vi "IMAQ-MWT (FPGA) without PA.vi"() -> ()   [LabVIEW 2015]
uses:
  Modules/Common/Controls (FPGA)/Camera Tap Configuration.ctl
  Modules/Common/Controls (FPGA)/Run Mode.ctl
  <vilib>/Platform/TimedLoop/XDataNode/timing_clust.ctl
  <vilib>/Platform/TimedLoop/XDataNode/nitl_modes.ctl
  <vilib>/Platform/TimedLoop/XDataNode/wakeup.ctl
  Modules/Common/Controls (FPGA)/CL Configuration.ctl
  Modules/Common/Controls (FPGA)/CL Signal Mapping.ctl
  Modules/Common/Controls (FPGA)/Pixel Bundle 40 Bytes.ctl
  <vilib>/rvi/eio/common/nirviEmuTemplateMethod_errors.vi
  <vilib>/rvi/Emulation/niFpgaSctlEmulationGetInTimedLoop.vi
  <vilib>/rvi/Emulation/niFpgaEmulationReportErrorSimple.vi
  <vilib>/rvi/Emulation/niFpgaGetClockAttributes.vi
  <vilib>/rvi/Emulation/niFpgaCriticalErrorInLSC.vi
  Modules/CL Data to Pixels/8 Tap 8-Bit.vi
  Modules/CL Data to Pixels/10 Tap 8-Bit.vi
  <vilib>/rvi/Emulation/niFpgaEmulationIsFPGAContextNoSignature.vi
  <vilib>/rvi/errors/niFpgaSetErrorForExecOnDevCompSimple.vi
  <vilib>/rvi/eio/common/nirviEmuReportErrorAndStop.vi
  <vilib>/rvi/DataTransferAndStorage/Container/Common/niFpgaContainerGetUniqueNameForEmu.vi
  <vilib>/rvi/FIFO/Fifo_Resource/nirvififoEmulationSetSize.vi
  <vilib>/rvi/FIFO/Fifo_Resource/nirviFifoEmulationQueueMgr.vi
  <instcachedir>/0/nirviFifoEmulationQueueMgr_E5CAEC123FF24DC58D834DCA3CDAA9B5.lvgen/nirviFifoEmulationQueueMgr_E5CAEC123FF24DC58D834DCA3CDAA9B5_008.vi
  <vilib>/rvi/FIFO/Fifo_Resource/nirvififoEmulationDetermineInputValidOut.vi
  <vilib>/rvi/FIFO/Fifo_Resource/nirvififoEmulationCreateLock.vi
  <vilib>/rvi/Emulation/niFpgaProcessEmulError.vi
  <vilib>/rvi/FIFO/Fifo_Resource/nirvififoEmulationObtainLock.vi
  <vilib>/rvi/FIFO/Fifo_Resource/nirvififoEmulationReleaseLock.vi
  <vilib>/rvi/occurrence/nirviWaitOnOccurrenceBase.vi
  <vilib>/rvi/errors/nirviReportUnexpectedCaseInternalError.vi
  <vilib>/rvi/errors/nirviReportUnexpectedCaseInternalError (U32).vi
  <instcachedir>/0/nirviFifoEmulationQueueMgr_E5CAEC123FF24DC58D834DCA3CDAA9B5.lvgen/nirviFifoEmulationQueueMgr_E5CAEC123FF24DC58D834DCA3CDAA9B5_004.vi
  <vilib>/Utility/error.llb/Clear Errors.vi
  <vilib>/rvi/interface/RandomDataEmulation/niFpgaRandomDataHandleErrors.vi
  <instcachedir>/0/nirviFifoEmulationQueueMgr_E5CAEC123FF24DC58D834DCA3CDAA9B5.lvgen/nirviFifoEmulationQueueMgr_E5CAEC123FF24DC58D834DCA3CDAA9B5_001.vi
  <vilib>/eio/EIONode/EIONode.xnode
  <vilib>/Platform/TimedLoop/XDataNode/XDataNode.xnode
  <vilib>/rvi/DataTransferAndStorage/Container/XNode/niFpgaContainer.xnode
  <vilib>/rvi/FIFO/Fifo_Resource/nirvififoEmulationWrite.vi
  <vilib>/rvi/FIFO/Fifo_Resource/nirvififoEmulationRead.vi
  <vilib>/rvi/interface/RandomDataEmulation/nirviRandomDataFpgaReadWriteTemplate.vi
  <vilib>/Platform/TimedLoop/XDataNode/XDNodeRunTimeDep.lvlib
panel:
  in  "Significant Angle":fxp<+,16,3>=0.0999755859375 format="%#_14g"
  in  "Mode":T1
  out "Frame Interval":u32=4294967295
  out "Frame #":u32
  in  "Image Height":u16=3072
  in  "Image Width":u16=3072
  out "PoCL Power Is On":bool
  in  "N Spline Points":fxp<+,8,8>=31.0
  in  "Clock Cycles Limit":u32=10000
  in  "Pixel Intensity":cluster{"Low":u8, "High":u8}={"Low"=100, "High"=255}
  out "DMA Timeout":bool
  in  "Cancel Acq":bool
  in  "Acquire":bool
  out "Acq In Progress":bool
  in  "Tap Configuration":T2
  in  "Initialize":bool=TRUE
  out "Initialized":bool=TRUE
  # "IMAQ - MWT"
  # "Camera Link Configuration"
  # "Acquisition Settings"
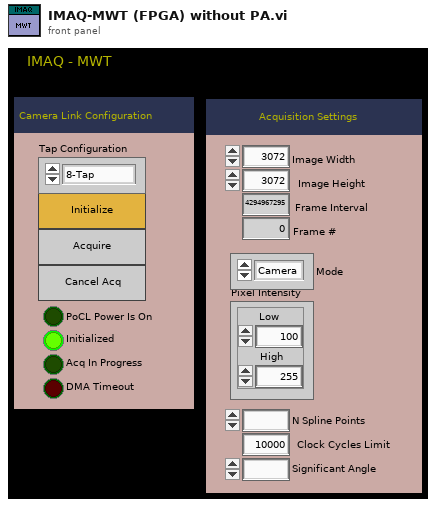
[diagram p1: front panel]
types:
  T1 = typedef "Run Mode.ctl" = enum16{"Camera", "Video (Raw)", "Video (DBDE)"}
  T2 = typedef "Camera Tap Configuration.ctl" = enum8{"8-Tap", "10-Tap"}
  T3 = typedef "CL Signal Mapping.ctl" = enum8{"Standard", "Basler 10-tap", "Vosskühler 10-tap"}
  T4 = typedef "CL Configuration.ctl" = enum8{"Base", "Medium", "Full"}
  T5 = typedef "XDNodeRunTimeDep.lvlib/timing_clust.ctl" = cluster{"Expected End [f-1]":u64, "Actual End [f-1]":u64, "Finished Late? [f-1]":bool, "Expected End [i-1]":u64, "Actual End [i-1]":u64, "Finished Late? [i-1]":bool, "Expected Start [i]":u64, "Actual Start [i]":u64, "Expected Start [f]":u64, "Actual Start [f]":u64, "Source Name":string, "Structure Name":string, "Period":i64, "Deadline":i64, "Offset":i64, "Start":i64, "Priority":i32, "Timeout":i32, "Mode":T6, "Wakeup Reason":T7, "Error":errorcluster, "Source Type":string, "Secondary Source Type":string, "Global End Time":u64, "Global Start Time":u64, "Frame Duration":u64, "Iteration Duration":u64, "Assigned CPU":i32, "I/O Scan Engine Mode":u32}
  T6 = typedef "XDNodeRunTimeDep.lvlib/nitl_modes.ctl" = enum32{"No Change", "Process missed periods, maintain original phase", "Discard missed periods, maintain original phase", "Process missed periods, ignore original phase", "Discard missed periods, ignore original phase"}
  T7 = typedef "XDNodeRunTimeDep.lvlib/wakeup.ctl" = enum32{"Normal", "Aborted", "Asynchronous wakeup", "Timing source error", "Timed loop error", "Timeout"}
  T8 = typedef "Pixel Bundle 40 Bytes.ctl" = cluster{"Pixel 1":u8, "Pixel 2":u8, "Pixel 3":u8, "Pixel 4":u8, "Pixel 5":u8, "Pixel 6":u8, "Pixel 7":u8, "Pixel 8":u8, "Pixel 9":u8, "Pixel 10":u8, "Pixel 11":u8, "Pixel 12":u8, "Pixel 13":u8, "Pixel 14":u8, "Pixel 15":u8, "Pixel 16":u8, "Pixel 17":u8, "Pixel 18":u8, "Pixel 19":u8, "Pixel 20":u8, "Pixel 21":u8, "Pixel 22":u8, "Pixel 23":u8, "Pixel 24":u8, "Pixel 25":u8, "Pixel 26":u8, "Pixel 27":u8, "Pixel 28":u8, "Pixel 29":u8, "Pixel 30":u8, "Pixel 31":u8, "Pixel 32":u8, "Pixel 33":u8, "Pixel 34":u8, "Pixel 35":u8, "Pixel 36":u8, "Pixel 37":u8, "Pixel 38":u8, "Pixel 39":u8, "Pixel 40":u8}
  T9 = cluster{"Enables Valid":bool, "Frame Valid":bool, "Line Valid":bool, "Data Valid":bool}
  T10 = cluster{"Pixel 0":u8, "Pixel 1":u8, "Pixel 2":u8, "Pixel 3":u8, "Pixel 4":u8, "Pixel 5":u8, "Pixel 6":u8, "Pixel 7":u8, "Pixel 8":u8, "Pixel 9":u8}
  T11 = cluster{"Pixel 0":u8, "Pixel 1":u8, "Pixel 2":u8, "Pixel 3":u8, "Pixel 4":u8, "Pixel 5":u8, "Pixel 6":u8, "Pixel 7":u8}
  T12 = cluster{"Pixel 1":u8, "Pixel 2":u8, "Pixel 3":u8, "Pixel 4":u8, "Pixel 5":u8, "Pixel 6":u8, "Pixel 7":u8, "Pixel 8":u8, "Pixel 9":u8, "Pixel 10":u8}
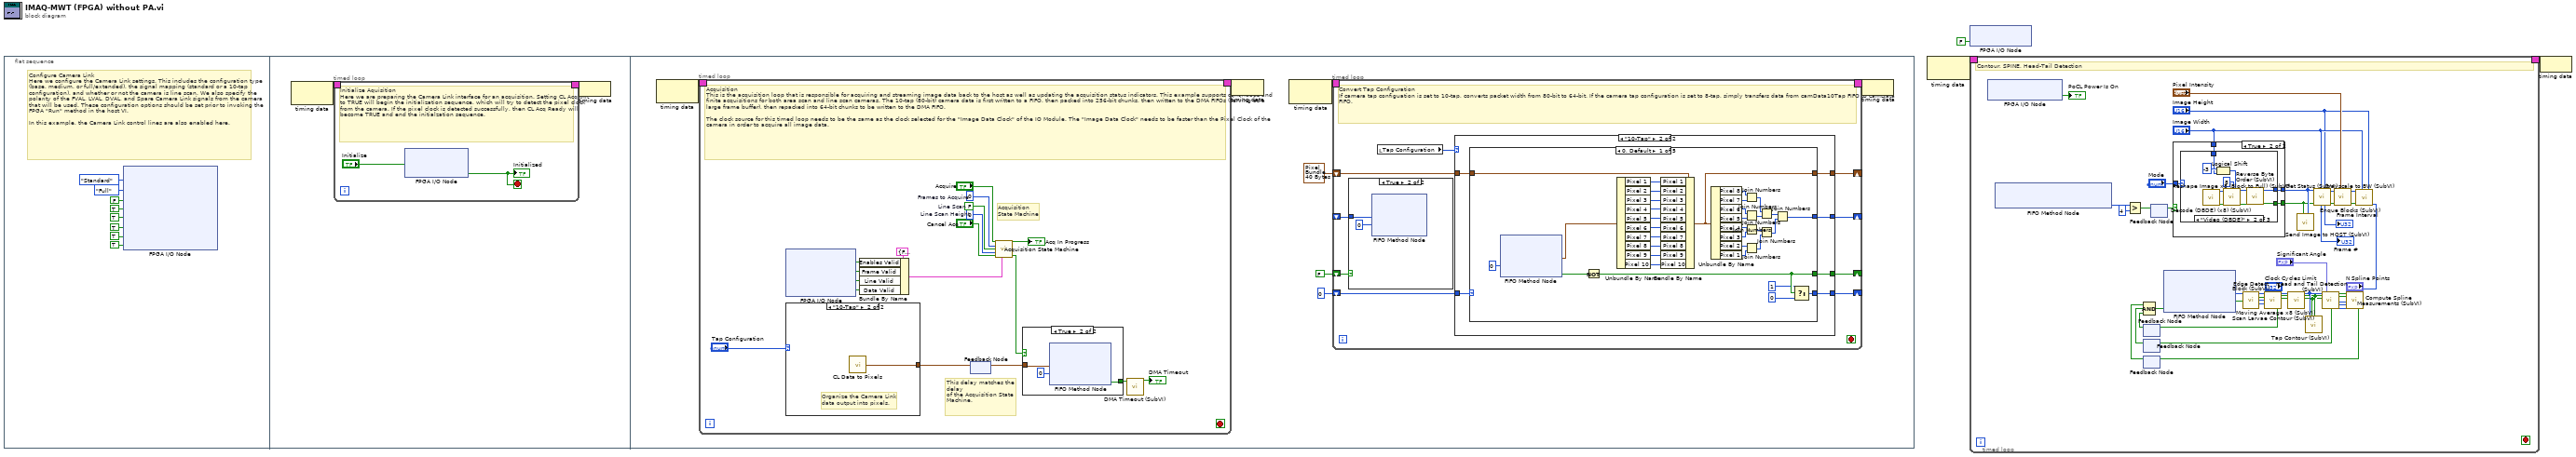
[diagram p0: block diagram]
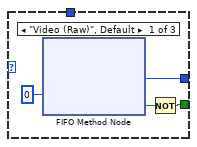
[diagram p3: hidden frame]
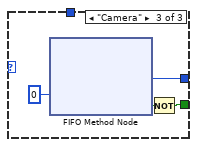
[diagram p4: hidden frame]
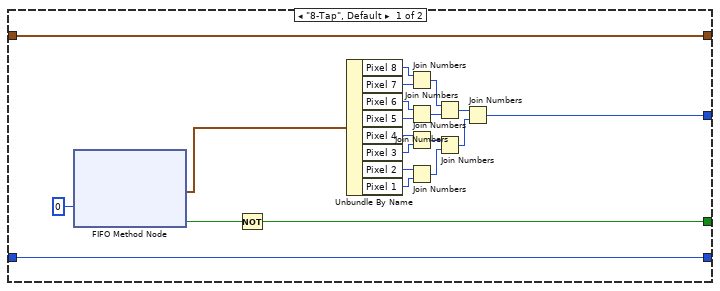
[diagram p6: hidden frame]
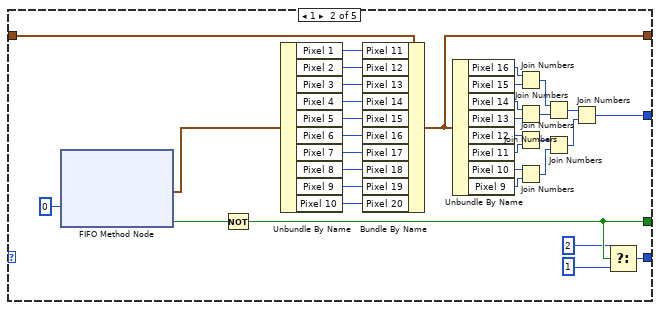
[diagram p7: hidden frame]
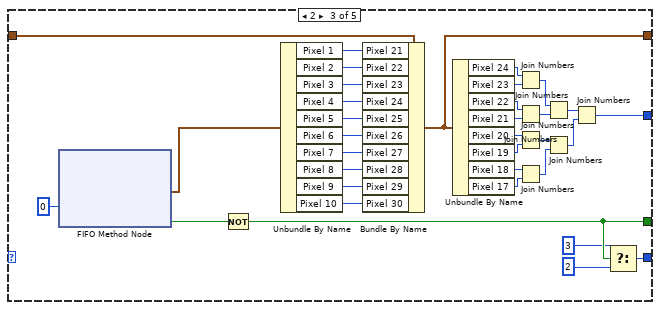
[diagram p8: hidden frame]
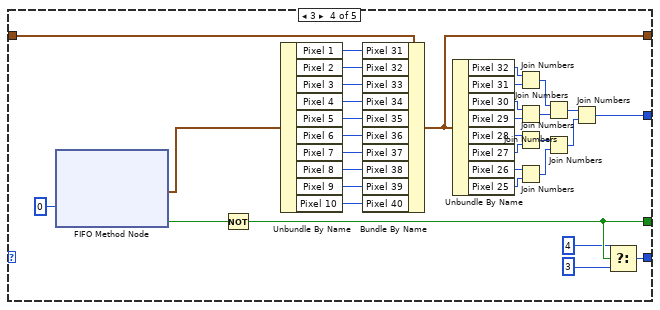
[diagram p9: hidden frame]
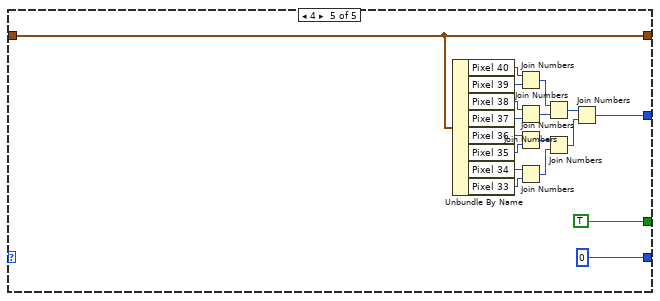
[diagram p10: hidden frame]
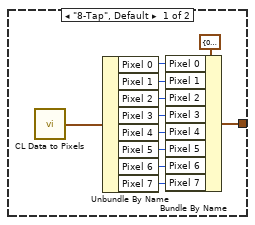
[diagram p11: hidden frame]
diagram:
  n1 = flat-sequence {
    frame #0 {
      # "Configure Camera Link\nHere we configure the Camera Link settings. This includes the configuration type (base, medium, or full/extended), the signal mapping (standard or a 10-tap configuration), and whether or not the camera is line scan. We also specify the polarity of the FVAL, LVAL, DVAL, and Spare Camera Link signals from the camera that will be used. These configuration options should be set prior to invoking the FPGA \"Run\" method in the host VI.\n\nIn this example, the Camera Link control lines are also enabled here."
      n2 = xnode "FPGA I/O Node"("CL Set Configuration"=CL_Signal_Mapping."Standard" ("Signal Mapping"), "CL Set Configuration"=CL_Configuration."Full" ("Configuration"), "CL Set Line Scan"=FALSE ("Line Scan"), "CL Set FVAL Active High"=TRUE ("FVAL Active High"), "CL Set LVAL Active High"=TRUE ("LVAL Active High"), "CL Set DVAL Active High"=TRUE ("DVAL Active High"), "CL Set Spare Active High"=TRUE ("Spare Active High"), "CL Control Enable"=TRUE ("IO Module\\CL Control Enable")) -> ()  [unwired: 8 in, 8 out]
    }
    frame #1 {
      n3 = node-c288() -> (w13:T5)  [unwired: 1 out]
      n4 = timed-loop {
        timing: w13 -> [_]
        timing-out: [_] -> w12
        stop <- w14 stop-if-true
        # "Initialize Aquisition\nHere we are preparing the Camera Link interface for an acquisition. Setting CL Acq Init to TRUE will begin the initialization sequence, which will try to detect the pixel clock from the camera. If the pixel clock is detected successfully, then CL Acq Ready will become TRUE and end the initialzation sequence."
        n5 = xnode "FPGA I/O Node"("CL Acq Init"="Initialize") -> ("CL Acq Ready"=w14:bool)  [unwired: 2 in, 2 out]
        "Initialized" <- w14
      }
      n6 = node-c288(w12) -> ()
    }
    frame #2 {
      n7 = node-c288() -> (w26:T5)  [unwired: 1 in]
      n8 = timed-loop {
        timing: w26 -> [_]
        timing-out: [_] -> w25
        stop <- _ stop-if-true
        w224 = FALSE  # Line Scan
        w225 = u32 0  # Line Scan Height
        w226 = u32 0  # Frames to Acquire
        # "This delay matches the delay\nof the Acquisition State Machine."
        # "Acquisition\nState Machine"
        # "Acquisition\nThis is the acquisition loop that is responsible for acquiring and streaming image data back to the host as well as updating the acquisition status indicators. This example supports continuous and finite acquisitions for both area scan and line scan cameras. The 10-tap (80-bit) camera data is first written to a FIFO, then packed into 256-bit chunks, then written to the DMA FIFOs (serving as a large frame buffer), then repacked into 64-bit chunks to be written to the DMA FIFO. \n\nThe clock source for this timed loop needs to be the same as the clock selected for the \"Image Data Clock\" of the IO Module. The \"Image Data Clock\" needs to be faster than the Pixel Clock of the camera in order to acquire all image data."
        n9 = xnode "FPGA I/O Node"() -> ("CL Output Valid"=w237:bool, "CL Frame Valid"=w236:bool, "CL Line Valid"=w235:bool, "CL Data Valid"=w233:bool)  [unwired: 4 in, 4 out]
        n10 = case shown="\"10-Tap\"" "Tap Configuration" {
          tunnel: [w241 w252] -> w229
          frame "8-Tap", Default {
            n11 = call-poly "CL Data to Pixels.vi"() -> ("Pixels"=w250:T11)  [unwired: 1 in]
            n12 = Unbundle By Name(w250) -> ("Pixel 0"=w249:u8, "Pixel 1"=w248:u8, "Pixel 2"=w247:u8, "Pixel 3"=w246:u8, "Pixel 4"=w245:u8, "Pixel 5"=w244:u8, "Pixel 6"=w243:u8, "Pixel 7"=w242:u8)
            n13 = Bundle By Name(cluster=T10 {"Pixel 0"=0, "Pixel 1"=0, "Pixel 2"=0, "Pixel 3"=0, "Pixel 4"=0, "Pixel 5"=0, "Pixel 6"=0, "Pixel 7"=0, "Pixel 8"=0, "Pixel 9"=0} ("Pixels"), "Pixel 0"=w249, "Pixel 1"=w248, "Pixel 2"=w247, "Pixel 3"=w246, "Pixel 4"=w245, "Pixel 5"=w244, "Pixel 6"=w243, "Pixel 7"=w242) -> (w241:T10)
          }
          frame "10-Tap" {
            # "Organize the Camera Link\ndata output into pixels."
            n14 = call-poly "CL Data to Pixels.vi"() -> ("Pixels"=w252:T10)  [unwired: 1 in]
          }
        }
        n15 = Bundle By Name(cluster=T9 {"Enables Valid"=FALSE, "Frame Valid"=FALSE, "Line Valid"=FALSE, "Data Valid"=FALSE} ("Enables"), "Enables Valid"=w237, "Frame Valid"=w236, "Line Valid"=w235, "Data Valid"=w233) -> (w234:T9)
        n16 = feedback-in #1(w229) -> ()
        n17 = feedback #1() -> (w230:T10)  [unwired: 1 in]
        n18 = call "Acquisition State Machine.vi"("Acquire"="Acquire", "Frames to Acquire"=w226, "Line Scan"=w224, "Line Scan Height"=w225, "Cancel Acq"="Cancel Acq", "Enables"=w234) -> ("Acq In Progress"=→"Acq In Progress":bool, "Capture Cycle"=w231:bool)  [unwired: 4 in, 4 out]
        n19 = case shown="True" w231 {
          tunnel: [_ w253] -> w227
          tunnel: w230 -> [_ w254]
          frame False {
          }
          frame True {
            n20 = xnode ("FIFO Method Node")("Element"=w254, "Timeout"=0) -> ("Timed Out?"=w253:bool)  [unwired: 1 in, 1 out]
          }
        }
        n21 = call "DMA Timeout (SubVI).vi"("Timeout"=w227) -> ("DMA Timeout"=→"DMA Timeout":bool)  [unwired: 10 in]
      }
      n22 = node-c288(w25) -> ()
      n23 = node-c288() -> (w24:T5)  [unwired: 1 in]
      n24 = timed-loop {
        timing: w24 -> [_]
        timing-out: [_] -> w23
        shift-right: [w33] -> _
        shift-left: u8 0 ("Timeout") -> [w34]
        shift-right: [w31] -> _
        shift-left: T8 {"Pixel 1"=0, "Pixel 2"=0, "Pixel 3"=0, "Pixel 4"=0, "Pixel 5"=0, "Pixel 6"=0, "Pixel 7"=0, "Pixel 8"=0, "Pixel 9"=0, "Pixel 10"=0, "Pixel 11"=0, "Pixel 12"=0, "Pixel 13"=0, "Pixel 14"=0, "Pixel 15"=0, "Pixel 16"=0, "Pixel 17"=0, "Pixel 18"=0, "Pixel 19"=0, "Pixel 20"=0, "Pixel 21"=0, "Pixel 22"=0, "Pixel 23"=0, "Pixel 24"=0, "Pixel 25"=0, "Pixel 26"=0, "Pixel 27"=0, "Pixel 28"=0, "Pixel 29"=0, "Pixel 30"=0, "Pixel 31"=0, "Pixel 32"=0, "Pixel 33"=0, "Pixel 34"=0, "Pixel 35"=0, "Pixel 36"=0, "Pixel 37"=0, "Pixel 38"=0, "Pixel 39"=0, "Pixel 40"=0} ("Data In") -> [w32]
        shift-right: [w30] -> _
        shift-left: _ -> [w27]
        shift-right: [w29] -> _
        shift-left: FALSE -> [w28]
        stop <- _ stop-if-true
        # "Convert Tap Configuration\nIf camera tap configuation is set to 10-tap, converts packet width from 80-bit to 64-bit. If the camera tap configuration is set to 8-tap, simply transfers data from camData10Tap FIFO to camData FIFO."
        n25 = case shown="True" w28 {
          tunnel: w27 -> [_ w37]
          frame False {
          }
          frame True {
            n26 = xnode ("FIFO Method Node")("Element"=w37, "Timeout"=0) -> ()  [unwired: 1 in, 2 out]
          }
        }
        n27 = local read "Tap Configuration"() -> (w35:T2)
        n28 = case shown="\"10-Tap\"" w35 {
          tunnel: [w44 w63] -> w29
          tunnel: [w43 w62] -> w30
          tunnel: w34 -> [w42 w64]
          tunnel: [w42 w61] -> w33
          tunnel: w32 -> [w41 w60]
          tunnel: [w41 w59] -> w31
          frame "8-Tap", Default {
            n29 = xnode ("FIFO Method Node")("Timeout"=0) -> ("Element"=w40:T12, "Timed Out?"=w39:bool)  [unwired: 1 in, 1 out]
            n30 = Not(x=w39) -> (.not. x?=w44:bool)
            n31 = Unbundle By Name(w40) -> ("Pixel 8"=w58:u8, "Pixel 7"=w57:u8, "Pixel 6"=w56:u8, "Pixel 5"=w55:u8, "Pixel 4"=w53:u8, "Pixel 3"=w54:u8, "Pixel 2"=w51:u8, "Pixel 1"=w52:u8)
            n32 = Join Numbers(hi=w58, lo=w57) -> ((hi.lo)=w49:u16)
            n33 = Join Numbers(hi=w56, lo=w55) -> ((hi.lo)=w50:u16)
            n34 = Join Numbers(hi=w53, lo=w54) -> ((hi.lo)=w48:u16)
            n35 = Join Numbers(hi=w51, lo=w52) -> ((hi.lo)=w47:u16)
            n36 = Join Numbers(hi=w49, lo=w50) -> ((hi.lo)=w46:u32)
            n37 = Join Numbers(hi=w48, lo=w47) -> ((hi.lo)=w45:u32)
            n38 = Join Numbers(hi=w46, lo=w45) -> ((hi.lo)=w43:u64)
          }
          frame "10-Tap" {
            n39 = case shown="0, Default" w64 {
              tunnel: [w82 w116 w150 w184 TRUE] -> w63
              tunnel: [w84 w118 w152 w186 w204] -> w62
              tunnel: [w83 w117 w151 w185 u8 0 ("Timeout")] -> w61
              tunnel: w60 -> [w79 w113 w147 w181 w203]
              tunnel: [w78 w112 w146 w180 w203] -> w59
              frame 0, Default {
                n40 = xnode ("FIFO Method Node")("Timeout"=0) -> ("Element"=w66:T12, "Timed Out?"=w67:bool)  [unwired: 1 in, 1 out]
                n41 = Not(x=w67) -> (.not. x?=w82:bool)
                n42 = Unbundle By Name(w66) -> ("Pixel 1"=w77:u8, "Pixel 2"=w76:u8, "Pixel 3"=w75:u8, "Pixel 4"=w74:u8, "Pixel 5"=w73:u8, "Pixel 6"=w72:u8, "Pixel 7"=w71:u8, "Pixel 8"=w70:u8, "Pixel 9"=w69:u8, "Pixel 10"=w68:u8)
                n43 = Bundle By Name(cluster=w79, "Pixel 1"=w77, "Pixel 2"=w76, "Pixel 3"=w75, "Pixel 4"=w74, "Pixel 5"=w73, "Pixel 6"=w72, "Pixel 7"=w71, "Pixel 8"=w70, "Pixel 9"=w69, "Pixel 10"=w68) -> (w78:T8)
                n44 = Unbundle By Name(w78) -> ("Pixel 8"=w98:u8, "Pixel 7"=w97:u8, "Pixel 6"=w96:u8, "Pixel 5"=w95:u8, "Pixel 4"=w93:u8, "Pixel 3"=w94:u8, "Pixel 2"=w91:u8, "Pixel 1"=w92:u8)
                n45 = Join Numbers(hi=w98, lo=w97) -> ((hi.lo)=w89:u16)
                n46 = Join Numbers(hi=w96, lo=w95) -> ((hi.lo)=w90:u16)
                n47 = Join Numbers(hi=w93, lo=w94) -> ((hi.lo)=w88:u16)
                n48 = Join Numbers(hi=w91, lo=w92) -> ((hi.lo)=w87:u16)
                n49 = Join Numbers(hi=w89, lo=w90) -> ((hi.lo)=w86:u32)
                n50 = Join Numbers(hi=w88, lo=w87) -> ((hi.lo)=w85:u32)
                n51 = Join Numbers(hi=w86, lo=w85) -> ((hi.lo)=w84:u64)
                n52 = Select(t=u8 1 ("Timeout"), s=w82, f=u8 0 ("Timeout")) -> (s? t:f=w83:u8)
              }
              frame 1 {
                n53 = xnode ("FIFO Method Node")("Timeout"=0) -> ("Element"=w101:T12, "Timed Out?"=w100:bool)  [unwired: 1 in, 1 out]
                n54 = Not(x=w100) -> (.not. x?=w116:bool)
                n55 = Unbundle By Name(w101) -> ("Pixel 1"=w111:u8, "Pixel 2"=w110:u8, "Pixel 3"=w109:u8, "Pixel 4"=w108:u8, "Pixel 5"=w107:u8, "Pixel 6"=w106:u8, "Pixel 7"=w105:u8, "Pixel 8"=w104:u8, "Pixel 9"=w103:u8, "Pixel 10"=w102:u8)
                n56 = Bundle By Name(cluster=w113, "Pixel 11"=w111, "Pixel 12"=w110, "Pixel 13"=w109, "Pixel 14"=w108, "Pixel 15"=w107, "Pixel 16"=w106, "Pixel 17"=w105, "Pixel 18"=w104, "Pixel 19"=w103, "Pixel 20"=w102) -> (w112:T8)
                n57 = Unbundle By Name(w112) -> ("Pixel 16"=w132:u8, "Pixel 15"=w131:u8, "Pixel 14"=w130:u8, "Pixel 13"=w129:u8, "Pixel 12"=w127:u8, "Pixel 11"=w128:u8, "Pixel 10"=w125:u8, "Pixel 9"=w126:u8)
                n58 = Join Numbers(hi=w132, lo=w131) -> ((hi.lo)=w123:u16)
                n59 = Join Numbers(hi=w130, lo=w129) -> ((hi.lo)=w124:u16)
                n60 = Join Numbers(hi=w127, lo=w128) -> ((hi.lo)=w122:u16)
                n61 = Join Numbers(hi=w125, lo=w126) -> ((hi.lo)=w121:u16)
                n62 = Join Numbers(hi=w123, lo=w124) -> ((hi.lo)=w120:u32)
                n63 = Join Numbers(hi=w122, lo=w121) -> ((hi.lo)=w119:u32)
                n64 = Join Numbers(hi=w120, lo=w119) -> ((hi.lo)=w118:u64)
                n65 = Select(t=u8 2 ("Timeout"), s=w116, f=u8 1 ("Timeout")) -> (s? t:f=w117:u8)
              }
              frame 2 {
                n66 = xnode ("FIFO Method Node")("Timeout"=0) -> ("Element"=w134:T12, "Timed Out?"=w135:bool)  [unwired: 1 in, 1 out]
                n67 = Not(x=w135) -> (.not. x?=w150:bool)
                n68 = Unbundle By Name(w134) -> ("Pixel 1"=w145:u8, "Pixel 2"=w144:u8, "Pixel 3"=w143:u8, "Pixel 4"=w142:u8, "Pixel 5"=w141:u8, "Pixel 6"=w140:u8, "Pixel 7"=w139:u8, "Pixel 8"=w138:u8, "Pixel 9"=w137:u8, "Pixel 10"=w136:u8)
                n69 = Bundle By Name(cluster=w147, "Pixel 21"=w145, "Pixel 22"=w144, "Pixel 23"=w143, "Pixel 24"=w142, "Pixel 25"=w141, "Pixel 26"=w140, "Pixel 27"=w139, "Pixel 28"=w138, "Pixel 29"=w137, "Pixel 30"=w136) -> (w146:T8)
                n70 = Unbundle By Name(w146) -> ("Pixel 24"=w166:u8, "Pixel 23"=w165:u8, "Pixel 22"=w164:u8, "Pixel 21"=w163:u8, "Pixel 20"=w161:u8, "Pixel 19"=w162:u8, "Pixel 18"=w159:u8, "Pixel 17"=w160:u8)
                n71 = Join Numbers(hi=w166, lo=w165) -> ((hi.lo)=w157:u16)
                n72 = Join Numbers(hi=w164, lo=w163) -> ((hi.lo)=w158:u16)
                n73 = Join Numbers(hi=w161, lo=w162) -> ((hi.lo)=w156:u16)
                n74 = Join Numbers(hi=w159, lo=w160) -> ((hi.lo)=w155:u16)
                n75 = Join Numbers(hi=w157, lo=w158) -> ((hi.lo)=w154:u32)
                n76 = Join Numbers(hi=w156, lo=w155) -> ((hi.lo)=w153:u32)
                n77 = Join Numbers(hi=w154, lo=w153) -> ((hi.lo)=w152:u64)
                n78 = Select(t=u8 3 ("Timeout"), s=w150, f=u8 2 ("Timeout")) -> (s? t:f=w151:u8)
              }
              frame 3 {
                n79 = xnode ("FIFO Method Node")("Timeout"=0) -> ("Element"=w168:T12, "Timed Out?"=w169:bool)  [unwired: 1 in, 1 out]
                n80 = Not(x=w169) -> (.not. x?=w184:bool)
                n81 = Unbundle By Name(w168) -> ("Pixel 1"=w179:u8, "Pixel 2"=w178:u8, "Pixel 3"=w177:u8, "Pixel 4"=w176:u8, "Pixel 5"=w175:u8, "Pixel 6"=w174:u8, "Pixel 7"=w173:u8, "Pixel 8"=w172:u8, "Pixel 9"=w171:u8, "Pixel 10"=w170:u8)
                n82 = Bundle By Name(cluster=w181, "Pixel 31"=w179, "Pixel 32"=w178, "Pixel 33"=w177, "Pixel 34"=w176, "Pixel 35"=w175, "Pixel 36"=w174, "Pixel 37"=w173, "Pixel 38"=w172, "Pixel 39"=w171, "Pixel 40"=w170) -> (w180:T8)
                n83 = Unbundle By Name(w180) -> ("Pixel 32"=w200:u8, "Pixel 31"=w199:u8, "Pixel 30"=w198:u8, "Pixel 29"=w197:u8, "Pixel 28"=w195:u8, "Pixel 27"=w196:u8, "Pixel 26"=w193:u8, "Pixel 25"=w194:u8)
                n84 = Join Numbers(hi=w200, lo=w199) -> ((hi.lo)=w191:u16)
                n85 = Join Numbers(hi=w198, lo=w197) -> ((hi.lo)=w192:u16)
                n86 = Join Numbers(hi=w195, lo=w196) -> ((hi.lo)=w190:u16)
                n87 = Join Numbers(hi=w193, lo=w194) -> ((hi.lo)=w189:u16)
                n88 = Join Numbers(hi=w191, lo=w192) -> ((hi.lo)=w188:u32)
                n89 = Join Numbers(hi=w190, lo=w189) -> ((hi.lo)=w187:u32)
                n90 = Join Numbers(hi=w188, lo=w187) -> ((hi.lo)=w186:u64)
                n91 = Select(t=u8 4 ("Timeout"), s=w184, f=u8 3 ("Timeout")) -> (s? t:f=w185:u8)
              }
              frame 4 {
                n92 = Unbundle By Name(w203) -> ("Pixel 40"=w218:u8, "Pixel 39"=w217:u8, "Pixel 38"=w216:u8, "Pixel 37"=w215:u8, "Pixel 36"=w213:u8, "Pixel 35"=w214:u8, "Pixel 34"=w211:u8, "Pixel 33"=w212:u8)
                n93 = Join Numbers(hi=w218, lo=w217) -> ((hi.lo)=w209:u16)
                n94 = Join Numbers(hi=w216, lo=w215) -> ((hi.lo)=w210:u16)
                n95 = Join Numbers(hi=w213, lo=w214) -> ((hi.lo)=w208:u16)
                n96 = Join Numbers(hi=w211, lo=w212) -> ((hi.lo)=w207:u16)
                n97 = Join Numbers(hi=w209, lo=w210) -> ((hi.lo)=w206:u32)
                n98 = Join Numbers(hi=w208, lo=w207) -> ((hi.lo)=w205:u32)
                n99 = Join Numbers(hi=w206, lo=w205) -> ((hi.lo)=w204:u64)
              }
            }
          }
        }
      }
      n100 = node-c288(w23) -> ()
    }
  }
  n101 = node-c288() -> (w3:T5)  [unwired: 1 in]
  n102 = xnode "FPGA I/O Node"("PoCL Disable"=FALSE) -> ()  [unwired: 1 in, 1 out]
  n103 = timed-loop {
    timing: w3 -> [_]
    timing-out: [_] -> w2
    stop <- _ stop-if-true
    # "Contour, SPINE, Head-Tail Detection"
    n104 = xnode "FPGA I/O Node"() -> ("PoCL Power Is On"=→"PoCL Power Is On":bool)  [unwired: 1 in, 1 out]
    n105 = xnode ("FIFO Method Node")() -> ("Number of Elements to Write"=w285:u32)  [unwired: 1 in, 1 out]
    n106 = Greater?(x=w285, y=u32 4) -> (0:w289:bool)
    n107 = feedback #2() -> (w292:bool)  [unwired: 1 in]
    n108 = feedback #3() -> (w293:bool)  [unwired: 1 in]
    n109 = feedback #4() -> (w291:bool)  [unwired: 1 in]
    n110 = Compound Arithmetic op=AND(w291, w293, w292) -> (w284:bool)
    n111 = feedback-in #5(w289) -> ()
    n112 = feedback #5() -> (w288:bool)  [unwired: 1 in]
    n113 = xnode ("FIFO Method Node")("Ready for Output"=w284) -> ("Element"=w283:u8, "Output Valid"=w282:bool)  [unwired: 1 in, 1 out]
    n114 = case shown="True" w288 {
      tunnel: "Mode" -> [_ w308]
      tunnel: "Image Width" -> [_ w307]
      tunnel: [_ w306] -> w298
      tunnel: [_ w305] -> w268
      frame False {
      }
      frame True {
        n115 = case shown="\"Video (DBDE)\"" w308 {
          tunnel: [w312 w317 w325] -> w305
          tunnel: [w311 w318 w324] -> w306
          tunnel: w307 -> [_ w315 _]
          frame "Video (Raw)", Default {
            n116 = xnode ("FIFO Method Node")("Timeout"=0) -> ("Element"=w311:u64, "Timed Out?"=w310:bool)  [unwired: 1 in, 1 out]
            n117 = Not(x=w310) -> (.not. x?=w312:bool)
          }
          frame "Video (DBDE)" {
            n118 = call "Decode (DBDE) (x8) (SubVI).vi"() -> ("Output Valid"=w320:bool, "Data Out"=w319:u64)  [unwired: 10 in]
            n119 = Logical Shift(y=i16 -3, x=w315) -> (x << y=w314:u16)
            n120 = call "Reshape Image x8 (Block to Full) (SubVI).vi"("Pixel Data In"=w319, "Pixel In Valid?"=w320, "Block Size"=u16 8, "Image Width (/8)"=w314) -> ("Pixel Data Out"=w321:u64, "Pixel Out Valid?"=w317:bool)  [unwired: 14 in]
            n121 = call "Reverse Byte Order (SubVI).vi"("Data In"=w321) -> ("Data Out"=w318:u64)  [unwired: 10 in]
          }
          frame "Camera" {
            n122 = xnode ("FIFO Method Node")("Timeout"=0) -> ("Element"=w324:u64, "Timed Out?"=w323:bool)  [unwired: 1 in, 1 out]
            n123 = Not(x=w323) -> (.not. x?=w325:bool)
          }
        }
      }
    }
    n124 = call "Edge Detect Block (SubVI).vi"("Data In"=w283, "In Valid?"=w282) -> ("Data Out"=w281:u8, "Out Valid?"=w280:bool, "X Start"=w294:u16, "Y Start"=w295:u16)  [unwired: 10 in]
    n125 = call "Scan Larvae Contour (SubVI).vi"("Data In"=w281, "Input Valid?"=w280, "X Start"=w294, "Y Start"=w295, "Max. Scan Cycles"="Clock Cycles Limit") -> ("Ready for Input?"=w271:bool, "Boundary Point XY"=w277:u32, "Boundary Valid?"=w276:bool, "Scan End?"=w275:bool)  [unwired: 10 in, 1 out]
    n126 = feedback-in #2(w271) -> ()
    n127 = call "Moving Average x8 (SubVI).vi"("Point In"=w277, "Boundary Valid? In"=w276, "Scan End? In"=w275) -> ("Point Out"=w274:u32, "Boundary Valid? out"=w273:bool, "Scan End? Out"=w272:bool)  [unwired: 14 in]
    n128 = call "Send Image to HOST (SubVI).vi"("Pixel Data"=w298, "Input Valid"=w268) -> ()  [unwired: 10 in]
    n129 = call "Tap Contour (SubVI).vi"("Contour XY"=w274, "Complete?"=w272, "Input Valid?"=w273) -> ()  [unwired: 17 in]
    n130 = call "Get Status (SubVI).vi"("Image Height"="Image Height", "Image Width"="Image Width", "Input Valid?"=w268, "Pixel In"=w298) -> ("Pixel Valid?"=w302:bool, "Pixel Out"=w301:u64, "Frame Interval"=→"Frame Interval":u32, "Frame #"=→"Frame #":u32)  [unwired: 4 in]
    n131 = call "Head and Tail Detection (SubVI).vi"("Boundary Point XY"=w274, "Bondary Valid?"=w273, "Scan End?"=w272, "Significant Angle"="Significant Angle") -> ("Ready for Input?"=w270:bool, "Output Valid?"=w264:bool, "Skip Contour Analysis"=w265:bool, "Head Index"=w263:u16, "Tail Index"=w262:u16, "N Points"=w261:u16)  [unwired: 9 in, 1 out]
    n132 = feedback-in #3(w270) -> ()
    n133 = call "Grayscale to BW (SubVI).vi"("Threshold Range"="Pixel Intensity", "Input Valid"=w302, "Data In"=w301) -> ("Output Valid"=w286:bool, "Data Out"=w287:u64)  [unwired: 7 in]
    n134 = call "Enque Blocks (SubVI).vi"("Pixels In"=w287, "Image Width"="Image Width", "Image Height"="Image Height", "Input Valid?"=w286) -> ("HT Location"=w266:u64[])  [unwired: 11 in]
    n135 = call "Compute Spline Measurements (SubVI).vi"("Input Valid?"=w264, "Skip SPLINE?"=w265, "V1 (ID)"=w263, "V2 (ID)"=w262, "N Points"=w261, "N Spline Points"="N Spline Points", "HT Location"=w266) -> ("Ready for Input?"=w269:bool)  [unwired: 8 in, 4 out]
    n136 = feedback-in #4(w269) -> ()
  }
  n137 = node-c288(w2) -> ()
